vi "Test Get Cell Value.vi"(11 "Test Case In":refnum<class "Test Open Xml.lvclass">) -> (0 "error out":errorcluster, 3 "Test Case Out":refnum<class "Test Open Xml.lvclass">)   [LabVIEW 2021, in "Test Open Xml.lvclass"]
uses:
  Test Open Xml.lvclass
  C:/Program Files/National Instruments/LabVIEW 2025/vi.lib/Astemes/LUnit/Test Case.lvclass
  <vilib>/Astemes/LUnit/Test Case.lvclass/Test Case.ctl
  <vilib>/Astemes/LUnit/Core/LUnit Test Case/Private/Append Fail Result.vi
  <vilib>/Astemes/LUnit/Core/LUnit Test Case/Private/Append Pass Result.vi
  <vilib>/Astemes/LUnit/Core/LUnit Test Case/Private/Run In UI.vi
  <vilib>/Utility/error.llb/Clear Errors.vi
  Source/Open Xml.lvlib
  <vilib>/Astemes/LUnit/Test Case.lvclass
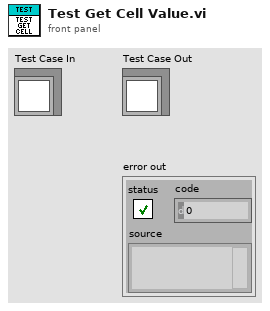
[diagram p1: front panel]
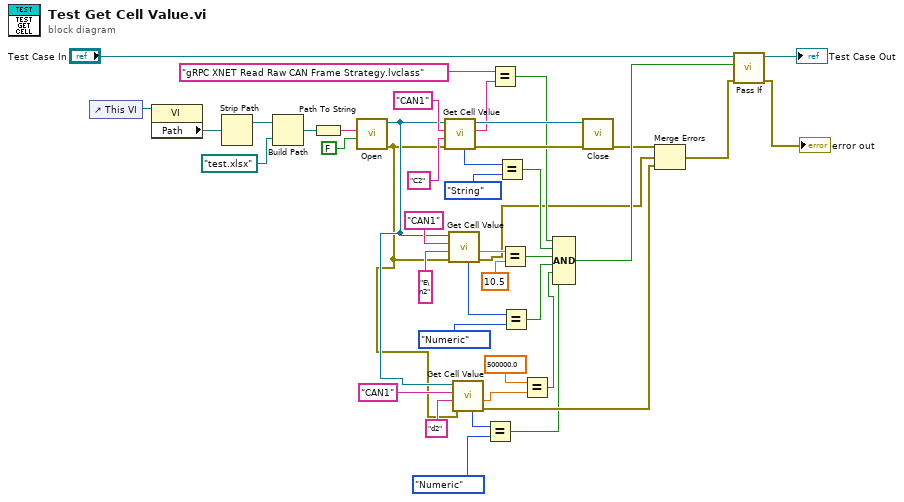
[diagram p0: block diagram]
diagram:
  n1 = control-ref of="This VI"() -> (w40:refnum<vi>)
  n2 = property class="VI"(reference=w40) -> ("Path"=w39:path)  [unwired: 1 in, 2 out]
  n3 = Strip Path(path=w39) -> (stripped path=w38:path)  [unwired: 1 out]
  n4 = Build Path(base path=w38, name or relative path=path "test.xlsx") -> (appended path=w36:path)
  n5 = Path To String(path=w36) -> (string=w35:string)
  n6 = call "Open.vi"("isEditable"=FALSE, "Path"=w35) -> ("error out"=w11:errorcluster, "SpreadsheetDocument"=w12:refnum<k24>)  [unwired: 8 in]
  n7 = call "Get Cell Value.vi"("error in"=w11, "Cell Address"="C2", "Sheet Name"="CAN1", "SpreadsheetDocument"=w12) -> ("error out"=w31:errorcluster, "Value String"=w28:string, "SpreadsheetDocument out"=w30:refnum<k24>, "Type"=w23:enum16{"String", "Numeric"})  [unwired: 3 in, 1 out]
  n8 = call "Get Cell Value.vi"("error in"=w11, "Cell Address"="E\n2", "Sheet Name"="CAN1", "SpreadsheetDocument"=w12) -> ("error out"=w9:errorcluster, "Value Numeric"=w24:dbl, "Type"=w21:enum16{"String", "Numeric"})  [unwired: 3 in, 2 out]
  n9 = call "Get Cell Value.vi"("error in"=w11, "Cell Address"="d2", "Sheet Name"="CAN1", "SpreadsheetDocument"=w12) -> ("error out"=w8:errorcluster, "Value Numeric"=w4:dbl, "Type"=w6:enum16{"String", "Numeric"})  [unwired: 3 in, 2 out]
  n10 = Equal?(x=w6, y=enum16{"String", "Numeric"}."Numeric") -> (x = y?=w1:bool)
  n11 = Equal?(x="gRPC XNET Read Raw CAN Frame Strategy.lvclass", y=w28) -> (x = y?=w16:bool)
  n12 = Equal?(x=w23, y=enum16{"String", "Numeric"}."String") -> (x = y?=w17:bool)
  n13 = Equal?(x=w24, y=10.5) -> (x = y?=w18:bool)
  n14 = Equal?(x=w21, y=enum16{"String", "Numeric"}."Numeric") -> (x = y?=w19:bool)
  n15 = Equal?(x=500000.0, y=w4) -> (x = y?=w2:bool)
  n16 = Compound Arithmetic op=AND(w16, w17, w18, w19, w2, w1) -> (w15:bool)
  n17 = call "Close.vi"("error in"=w31, "SpreadsheetDocument"=w30) -> ("error out"=w10:errorcluster)  [unwired: 9 in]
  n18 = Merge Errors(w10, w9, w8) -> (w7:errorcluster)
  n19 = call <vilib>:"Pass If.vi"("error in (no error)"=w7, "Pass?"=w15, "LUnit Test Case In"="Test Case In") -> ("error out"=→"error out":errorcluster, "LUnit Test Case Out"=→"Test Case Out":refnum<class "Test Open Xml.lvclass">)  [unwired: 7 in]
